vi "Write Listened To Msg.vi"(10 "Listened To Msg":bool, 11 "TEMPLATE Actor in":refnum<class "TEMPLATE Actor.lvclass">) -> (3 "TEMPLATE Actor out":refnum<class "TEMPLATE Actor.lvclass">)   [LabVIEW 2025, in "_Template.lvlib" / "Templates.lvlib" / "TEMPLATE Actor.lvlib" / "TEMPLATE Actor.lvclass"]
uses:
  TEMPLATE Actor.lvclass
  TEMPLATE Actor.lvclass/TEMPLATE Actor.ctl
  jettl/jettl/Actor/Actor.lvclass
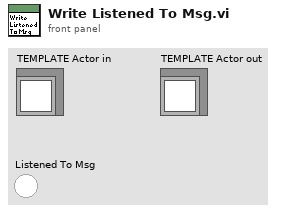
[diagram p1: front panel]
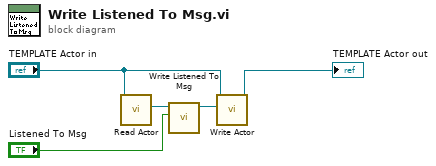
[diagram p0: block diagram]
diagram:
  n1 = call-dynamic "Read Actor.vi"("TEMPLATE Actor in"="TEMPLATE Actor in") -> ("Actor"=w3:refnum<class "Actor.lvclass">)  [unwired: 10 in]
  n2 = call-dynamic "Write Listened To Msg.vi"("Listened To Msg"="Listened To Msg", "Actor in"=w3) -> ("Actor out"=w1:refnum<class "Actor.lvclass">)  [unwired: 9 in]
  n3 = call-dynamic "Write Actor.vi"("Actor"=w1, "TEMPLATE Actor in"="TEMPLATE Actor in") -> ("TEMPLATE Actor out"=→"TEMPLATE Actor out":refnum<class "TEMPLATE Actor.lvclass">)  [unwired: 9 in]
